vi "Teleop.vi"(10 "Match Info":T1={"Autonomous Elapsed Seconds"=0.0, "TeleOp Elapsed Seconds"=0.0, "Disabled Elapsed Seconds"=0.0, "Visited Autonomous"=FALSE, "Visited TeleOp"=FALSE, "Visited Disabled"=FALSE, "Autonomous Settings"={"Autonomous Style"=enum."Independent", "VI Refnum"=refnum}}, 11 "Call Context":T2) -> ()   [LabVIEW 2013]
doc: "This VI is called for each TeleOp packet received from the DS where the robot is not disabled. It is often used to read from the joysticks and update I/O or to update setpoints for timed control loops. It should complete and return within 20 milliseconds or it may miss DS packets."
uses:
  <vilib>/Rock Robotics/WPI/DriverStation/WPI_DriverStationDerivedRobotMode.ctl
  <vilib>/Rock Robotics/WPI/DriverStation/WPI_DriverStationMatch Info.ctl
  RefnameEnum.ctl
  Robot Global Data.vi
  <vilib>/Rock Robotics/WPI/Joystick/WPI_JoystickGetSetRefNum.vi
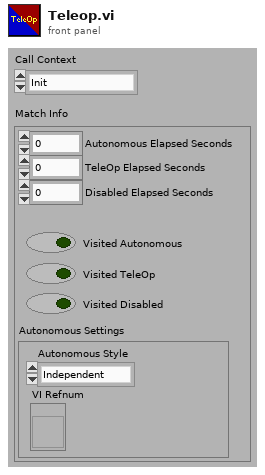
[diagram p1: front panel]
types:
  T1 = typedef "WPI_DriverStationMatch Info.ctl" = cluster{"Autonomous Elapsed Seconds":dbl, "TeleOp Elapsed Seconds":dbl, "Disabled Elapsed Seconds":dbl, "Visited Autonomous":bool, "Visited TeleOp":bool, "Visited Disabled":bool, "Autonomous Settings":cluster{"Autonomous Style":enum16{"Iterative", "Independent"}, "VI Refnum":refnum<vi>}}
  T2 = typedef "WPI_DriverStationDerivedRobotMode.ctl" = enum16{"Init", "Execute", "Stop"}
  T3 = typedef "RefnameEnum.ctl" = enum16{"TankDrive", "Controller1", "Controller2", "SonicShifter", "Compressor"}
  T4 = typedef "WPI_JoystickDevRef.ctl" = cluster{"Device":T5}
  T5 = typedef "WPI_JoystickDeviceEnum.ctl" = enum16{"USB 1", "USB 2", "USB 3", "USB 4", "Kinect 1", "Kinect 2"}
  T6 = typedef "WPI_JoystickButtonState.ctl" = cluster{"Button 1":bool, "Button 2":bool, "Button 3":bool, "Button 4":bool, "Button 5":bool, "Button 6":bool, "Button 7":bool, "Button 8":bool, "Button 9":bool, "Button 10":bool, "Button 11":bool, "Button 12":bool}
  T7 = cluster{"axis 1 (x)":dbl, "axis 2 (y)":dbl, "axis 3 (throttle)":dbl, "axis 4":dbl, "axis 5":dbl, "axis 6":dbl}
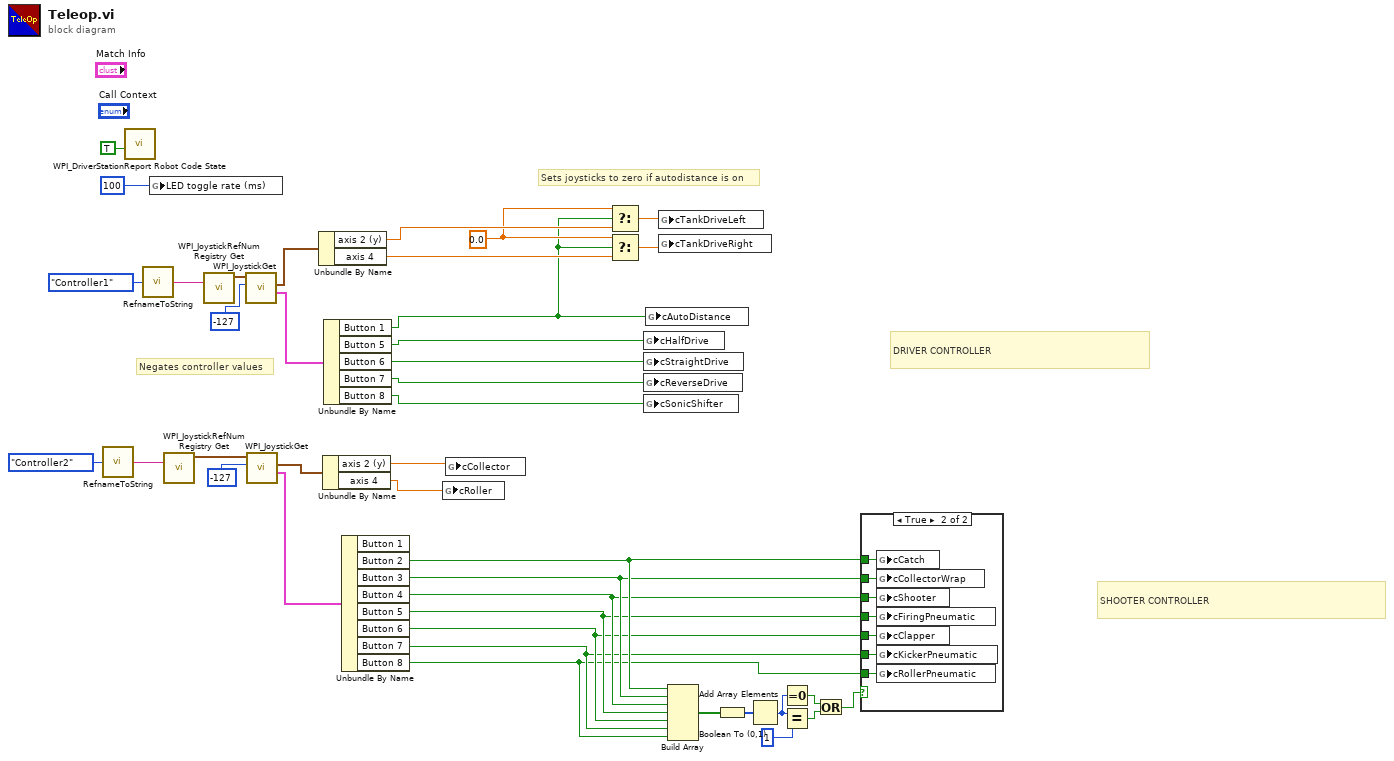
[diagram p0: block diagram]
diagram:
  w16 = 0.0 ("t")
  # "Sets joysticks to zero if autodistance is on"
  # "SHOOTER CONTROLLER"
  # "DRIVER CONTROLLER"
  # "Negates controller values"
  n1 = call "RefnameToString.vi"("Enum"=RefnameEnum."Controller2") -> ("Refname"=w27:string)
  n2 = call <vilib>:"WPI_DriverStationReport Robot Code State.vi"("TeleOp"=TRUE ("Autonomous")) -> ()  [unwired: 10 in, 1 out]
  n3 = call "RefnameToString.vi"("Enum"=RefnameEnum."Controller1") -> ("Refname"=w36:string)
  n4 = global write "Robot Global Data.vi" "LED toggle rate (ms)"(u32 100 ("LED ms toggle rate")) -> ()
  n5 = call <vilib>:"WPI_JoystickRefNum Registry Get.vi"("refnum name"=w27) -> ("JoystickDevRef"=w25:T4)  [unwired: 1 in, 9 out]
  n6 = call <vilib>:"WPI_JoystickRefNum Registry Get.vi"("refnum name"=w36) -> ("JoystickDevRef"=w38:T4)  [unwired: 1 in, 9 out]
  n7 = call <vilib>:"WPI_JoystickGet.vi"("Scaler"=i8 -127, "JoystickDevRef"=w38) -> ("Buttons"=w33:T6, "Axes"=w34:T7)  [unwired: 4 out]
  n8 = call <vilib>:"WPI_JoystickGet.vi"("Scaler"=i8 -127, "JoystickDevRef"=w25) -> ("Buttons"=w23:T6, "Axes"=w24:T7)  [unwired: 4 out]
  n9 = Unbundle By Name(w34) -> ("axis 2 (y)"=w17:dbl, "axis 4"=w18:dbl)
  n10 = Unbundle By Name(w24) -> ("axis 2 (y)"=w22:dbl, "axis 4"=w21:dbl)
  n11 = Unbundle By Name(w33) -> ("Button 1"=w15:bool, "Button 5"=w32:bool, "Button 6"=w31:bool, "Button 7"=w29:bool, "Button 8"=w30:bool)
  n12 = Unbundle By Name(w23) -> ("Button 2"=w11:bool, "Button 3"=w10:bool, "Button 4"=w9:bool, "Button 5"=w8:bool, "Button 6"=w7:bool, "Button 7"=w6:bool, "Button 8"=w5:bool)  [unwired: 1 out]
  n13 = global write "Robot Global Data.vi" "cRoller"(w21) -> ()
  n14 = global write "Robot Global Data.vi" "cCollector"(w22) -> ()
  n15 = Select(t=w16, s=w15, f=w17) -> (s? t:f=w20:dbl)
  n16 = Select(t=w16, s=w15, f=w18) -> (s? t:f=w19:dbl)
  n17 = global write "Robot Global Data.vi" "cHalfDrive"(w32) -> ()
  n18 = global write "Robot Global Data.vi" "cStraightDrive"(w31) -> ()
  n19 = global write "Robot Global Data.vi" "cReverseDrive"(w29) -> ()
  n20 = global write "Robot Global Data.vi" "cSonicShifter"(w30) -> ()
  n21 = global write "Robot Global Data.vi" "cAutoDistance"(w15) -> ()
  n22 = global write "Robot Global Data.vi" "cTankDriveLeft"(w20) -> ()
  n23 = global write "Robot Global Data.vi" "cTankDriveRight"(w19) -> ()
  n24 = Build Array(w11, w10, w9, w8, w7, w6, w5) -> (w12:bool[])
  n25 = Boolean To (0,1)(Boolean=w12) -> (0, 1=w13:i16[])
  n26 = Add Array Elements(numeric array=w13) -> (sum=w4:i16)
  n27 = Equal To 0?(x=w4) -> (x = 0?=w3:bool)
  n28 = Equal?(x=w4, y=i16 1) -> (x = y?=w2:bool)
  n29 = Or(x=w3, y=w2) -> (x .or. y?=w1:bool)
  n30 = case shown="True" w1 {
    tunnel: w11 -> [_ w47]
    tunnel: w10 -> [_ w46]
    tunnel: w9 -> [_ w45]
    tunnel: w8 -> [_ w44]
    tunnel: w7 -> [_ w43]
    tunnel: w6 -> [_ w42]
    tunnel: w5 -> [_ w41]
    frame False {
    }
    frame True {
      n31 = global write "Robot Global Data.vi" "cCatch"(w47) -> ()
      n32 = global write "Robot Global Data.vi" "cCollectorWrap"(w46) -> ()
      n33 = global write "Robot Global Data.vi" "cShooter"(w45) -> ()
      n34 = global write "Robot Global Data.vi" "cFiringPneumatic"(w44) -> ()
      n35 = global write "Robot Global Data.vi" "cClapper"(w43) -> ()
      n36 = global write "Robot Global Data.vi" "cKickerPneumatic"(w42) -> ()
      n37 = global write "Robot Global Data.vi" "cRollerPneumatic"(w41) -> ()
    }
  }
